vi "Dashboard Main.vi"() -> ()   [LabVIEW 2015]
uses:
  Auton Defenses Enum.ctl
  AutoStatesTypeDef.ctl
  <vilib>/Utility/miscctls.llb/LVRowAndColumnTypeDef.ctl
  <vilib>/event_ctls.llb/eventvkey.ctl
  <vilib>/Rock Robotics/WPI/Dashboard/WPI_DashboardLogging Global.vi
  <vilib>/Rock Robotics/Network Tables/NT Read Numeric Array.vi
  <vilib>/Rock Robotics/Network Tables/NT Write Boolean.vi
  <vilib>/Rock Robotics/Network Tables/NT Read Boolean.vi
  <vilib>/Rock Robotics/Network Tables/NT Write Numeric Array.vi
  <vilib>/Utility/config.llb/Write Key (String).vi
  <vilib>/Utility/config.llb/Write Key (I32).vi
  <vilib>/Utility/config.llb/NI_LVConfig.lvlib
panel:
  in  "End Point 2":cluster{"X":i32, "Y":i32}={"X"=158, "Y"=0}
  in  "Start Point 2":cluster{"X":i32, "Y":i32}={"X"=158, "Y"=240}
  in  "End Point":cluster{"X":i32, "Y":i32}={"X"=320, "Y"=120}
  in  "Start Point":cluster{"X":i32, "Y":i32}={"X"=0, "Y"=120}
  in  "Vision":u16(ring) items=["Camera Off", "USB Camera SW", "USB Camera HW", "IP Camera"]
  out "Detected Targets":T1(array[cluster]) {"Normalized Rect"."Numeric 5" format="%#_2g"; "Normalized Rect"."Numeric 3" format="%#_2g"; "Normalized Rect"."Numeric 2" format="%#_2g"; "Normalized Rect"."Numeric" format="%#_2g"}
  in  "TCP":refnum<k5>
  in  "Rec Mode":enum32{"Stop", "Record", "Playback"}(radio)
  out "Camera IP":string
  out "Image Message":string="Timeout in Camera Communications"
  in  "Dashboard Tab":T2(tab)
  out "Shooter at Speed":bool
  in  "Right Compensation":dbl
  in  "Left Compensation":dbl
  out "Rear Camera On?":bool
  out "Drive Shift":string
  out "Gyro Angle":dbl
  out "Drive Mode":string
  out "Shooter Speed":dbl
  out "Shooter Setpoint":dbl
  out "Hanging Pin Status":string
  out "Ball on Board?":bool
  in  "Defense":T3
  in  "Position":T4(ring)
  in  "Enable Vision?":bool
  out "Shooter Active?":bool
  in  "Gyro Reset":bool
  out "Acquiring?":bool
  out "Auton Current State":T5
  in  "Auton Shoot":bool
  in  "Select Auto":string(combo)
  out "NT Connection":bool
  in  "Camera Settings":T6={"Frame Rate"=30, "Compression"=30, "Size"=1} {"Frame Rate" scale=1.0..30.0; "Size" items=["640x480", "320x240", "160x120"]}
  out "MotorChart R":cluster{"Numeric":dbl, "Numeric":dbl}(graph)
  out "MotorChart L":T7(graph)
  out "MotorSliders R":cluster{"MotorSlide1":dbl, "MotorSlide2":dbl} {"MotorSlide2" scale=-1.0..1.0 scale format="%#_2e"; "MotorSlide1" scale=-1.0..1.0 scale format="%#_2e"}
  out "MotorSliders L":T8 {"MotorSlide4 2" scale=0.0..14.0 scale format="%#_2e"; "MotorSlide2" scale=-1.0..1.0 scale format="%#_2e"; "MotorSlide1" scale=-1.0..1.0 scale format="%#_2e"}
  out "Gyro":dbl(knob) scale=0.0..360.0
  out "JS1 Z":dbl(slide) scale=-1.0..1.0 scale format="%#_2e"
  out "JS1 Graph":cluster{"X":dbl, "Y":dbl}[](graph)
  out "JS1 Buttons":T9
  out "JS2 Z":dbl(slide) scale=-1.0..1.0 scale format="%#_2e"
  out "JS2 Graph":cluster{"X":dbl, "Y":dbl}[](graph)
  out "JS2 Buttons":T9
  out "Mode":T10(ring)=enum."Auto Disabled"
  in  "DB Camera Config":bool
  out "fps":dbl format="%#.1g"
  out "Mbps":dbl format="%#.1g"
  out "Mbps LED":bool
  in  "DB/String 9":string
  in  "DB/String 8":string
  in  "DB/String 7":string
  in  "DB/String 6":string
  in  "DB/String 5":string
  in  "DB/String 4":string
  in  "DB/String 3":string
  in  "DB/String 2":string
  in  "DB/String 1":string
  in  "DB/String 0":string
  in  "DB/Slider 0":dbl(slide) scale=0.0..5.0
  in  "DB/Slider 1":dbl(slide) scale=0.0..5.0
  in  "DB/Slider 2":dbl(slide) scale=0.0..5.0
  in  "DB/Slider 3":dbl(slide) scale=0.0..5.0
  out "DB/LED 3":bool
  out "DB/LED 2":bool
  out "DB/LED 1":bool
  out "DB/LED 0":bool
  in  "DB/Button 3":bool
  in  "DB/Button 2":bool
  in  "DB/Button 1":bool
  in  "DB/Button 0":bool caption="New Name"
  in  "Shooter Control":bool=TRUE
  in  "Top Wheel Speed Multiplier":dbl=0.8
  in  "Beater Bar Speed":dbl=0.75
  in  "LED Color":T11={"Hue"={77.0, 147.0}, "Sat"={140.0, 255.0}, "Val"={146.0, 255.0}} {"Hue" scale=0.0..255.0 scale format="%#_3g"}
  out "Target X Value":dbl
  in  "Shooter Power":dbl=0.5 step=0.01
  out "Shooter Speed (RPS)":dbl
  in  "Shooter Setpoint (RPS)":dbl=49.0 step=0.01
  in  "Shooter Wait (Seconds)":dbl=0.75 step=0.01
  out "Shooter Speed Top (RPS)":dbl
  in  "Test Slider":dbl(slide) scale=0.0..100.0 scale format="%#_3g"
  in  "On/Off":bool caption="Solenoid"
  in  "Test Name":u16(ring) items=["Select the test to run..."]
  in  "Test Tree":string(tree)
  in  "Motor":cluster{"Value":dbl, "Enable":bool} {"Value" scale=-1.0..1.0 scale format="%#_3g"}
  out "Progress":T12 {"Test Progress" scale=0.0..100.0}
  in  "Rev/Fwd":cluster{"Forward":bool, "Reverse":bool}
  in  "Test Ring":u16(ring) items=["Monochrome", "Color"]
  out "Cmd Status":string
  in  "Execute Command":bool
  in  "Command Params":string[][](table)
  in  "Command Selection":i32(listbox)
  in  "CheckList":i32(listbox)
  out "Tree":string(tree)
  out "Background":bool
  out "Unmasked Image":T13(plugin-control)
  # "Adds to specified,\nsubtracts from other(-1 to 1)"
  # "Left"
  # "Front"
  # "Right"
  # "Battery"
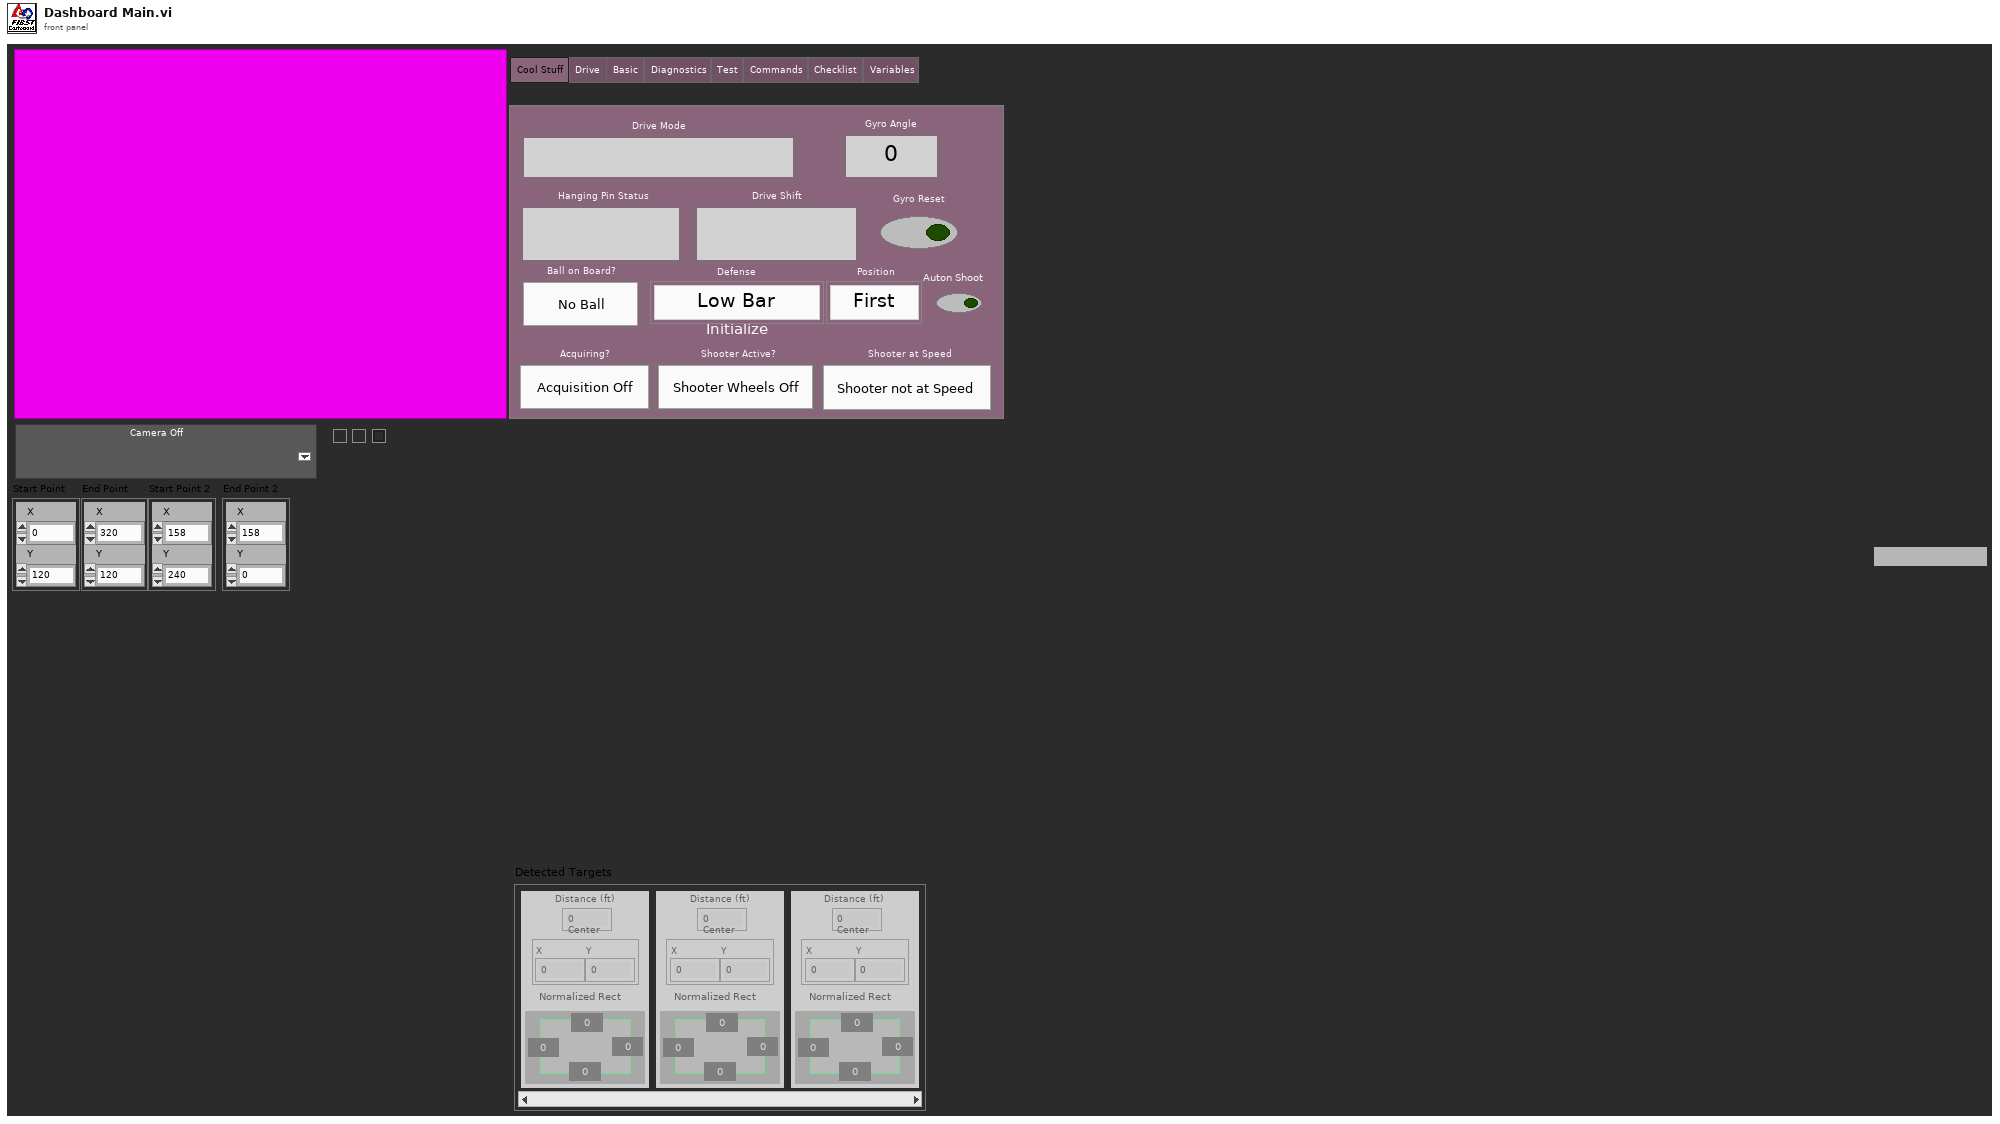
[diagram p1: front panel]
types:
  T1 = cluster{"Distance (ft)":dbl, "Center":cluster{"X":dbl, "Y":dbl}, "Normalized Rect":cluster{"Numeric":dbl, "Numeric 2":dbl, "Numeric 3":dbl, "Numeric 5":dbl}}[]
  T2 = enum32{"Cool Stuff", "Drive", "Basic", "Diagnostics", "Test", "Commands", "Checklist", "Variables"}
  T3 = typedef "Auton Defenses Enum.ctl" = enum16{"Low Bar", "None", "Portcullis", "CDF", "Moat", "Ramparts", "Drawbridge", "Sally Port", "Rock Wall", "Reach", "Spy Bot", "Rough Terrain"}
  T4 = enum16{"First", "Second", "Third", "Fourth", "Fifth"}
  T5 = typedef "AutoStatesTypeDef.ctl" = enum16{"Initialize", "Line up to shoot", "Align robot", "Drive to goal", "Lower Arms", "Raise Arms", "Drive to defense", "Cross defense", "Turn towards goal", "Shoot", "Retreat", "Stop"}
  T6 = cluster{"Frame Rate":i32, "Compression":i32, "Size":u16}
  T7 = cluster{"Numeric":dbl, "Numeric":dbl, "Battery V":dbl}
  T8 = cluster{"MotorSlide1":dbl, "MotorSlide2":dbl, "MotorSlide4 2":dbl}
  T9 = cluster{bool, bool, bool, bool, bool, bool, bool, bool, bool, bool, bool, bool}
  T10 = enum8{"Tele-Op Disabled", "Tele-Op Enabled", "Auto Disabled", "Auto Enabled", "Test Disabled", "Test Enabled", "Disconnected", "No Code", "E-Stop"}
  T11 = cluster{"Hue":cluster{dbl, dbl}, "Sat":cluster{dbl, dbl}, "Val":cluster{dbl, dbl}}
  T12 = cluster{"Test Progress":u8, "Test Progress Text":string}
  T13 = typedef "IMAQ Image.ctl" = refnum<image>
  T14 = cluster{"IDs":cluster{"RPC field ID":u16, "Unique ID":u16}, "String":string}
  T15 = enum32{"Drive", "Basic", "Custom", "Test", "Checklist", "Variables"}
  T16 = typedef "Image Type" = u32
  T17 = cluster{"Unmasked Image":refnum<vi>, "Dashboard Tab":refnum<vi>, "Background":refnum<vi>, "Vision":refnum<vi>, "Rec Mode":refnum<vi>, "Test Slider":refnum<vi>, "On/Off ":refnum<vi>, "Test Ring":refnum<vi>, "Rev/Fwd":refnum<vi>, "Test Name":refnum<vi>, "Motor":refnum<vi>, "Progress":refnum<vi>, "CheckList":refnum<vi>, "Tree":refnum<vi>, "Test Tree":refnum<vi>, "Command Params":refnum<vi>, "Command Selection":refnum<vi>, "Execute Command":refnum<vi>, "Cmd Status":refnum<vi>}
  T18 = typedef "NI_LVConfig.lvlib/Config Data RefNum.ctl" = refnum<k1>
  T19 = cluster{"Distance (ft)":dbl, "Center":cluster{dbl, dbl}, "Normalized Rect":cluster{"Numeric":dbl, "Numeric 2":dbl, "Numeric 3":dbl, "Numeric 5":dbl}}[]
  T20 = cluster{"Error Strings":string, "Disable Counts":cluster{u16, u16}, "Rail Faults":cluster{u16, u16, u16}, "Robot IP":string, "DB Mode":u8, "Event Info":cluster{"Name":string, "Type":u8, "Number":u16, "Replay":u8}, "Camera Addr":string}
  T21 = cluster{"Storage":cluster{"Disk Free":u64, "RAM Block":u32, "RAM free":u32}, "CPU Utilization":cluster{"CPU % ISR":sgl, "CPU % Time Crit":sgl, "CPU % Timed Str":sgl, "CPU % High":sgl, "CPU % Above":sgl, "CPU % Normal":sgl, "CPU % Low":sgl}, "CAN":cluster{"% Bus Utilization":sgl, "Bus Off Cnt":u32, "TX_FIFO Full Cnt":u32, "Receive Error Cnt":u8, "Transmit Error Cnt":u8}, "HID":cluster{"HID Outputs":u32, "Rumble Low":u16, "Rumble High":u16}[]}
  T22 = cluster{"Status bits":cluster{"Test Mode":bool, "Autonomous":bool, "Enabled":bool, "Code Start":bool, "Brownout":bool, "Reserved 2":bool, "Reserved 3":bool, "E-Stop":bool}, "Code Trace":cluster{"Disabled":bool, "TeleOp":bool, "Auto":bool, "Test":bool}, "Controller Type":enum16{"unknown", "cRIO", "roboRio"}, "Code?":enum16{"unknown", "noCode", "code"}, "Battery V":dbl}
  T23 = cluster{"Control Bits":cluster{"TestMode":bool, "Autonomous":bool, "Enabled":bool, "FMS Present":bool, bool, bool, bool, "E-Stop":bool}, "Team Station ":u8, "Countdown":sgl, "Joystick Values":cluster{"Axes":dbl[], "Buttons":bool[], "POVs":i16[]}[]}
  T24 = cluster{"Axes":dbl[], "Buttons":bool[], "POVs":i16[]}[]
  T25 = cluster{"Distance (ft)":dbl, "Center":cluster{"X":dbl, "Y":dbl}, "Normalized Rect":cluster{"Numeric":dbl, "Numeric 2":dbl, "Numeric 3":dbl, "Numeric 5":dbl}}
  T26 = cluster{"Axes":dbl[], "Buttons":bool[], "POVs":i16[]}
  T27 = cluster{"Buttons[0]":bool, "Buttons[1]":bool, "Buttons[2]":bool, "Buttons[3]":bool, "Buttons[4]":bool, "Buttons[5]":bool, "Buttons[6]":bool, "Buttons[7]":bool, "Buttons[8]":bool, "Buttons[9]":bool, "Buttons[10]":bool, "Buttons[11]":bool}
  T28 = cluster{"Operation":enum16{"Update", "Clear"}, "Color Box":u32}[]
  T29 = typedef "eventvkey.ctl" = enum16{"ASCII", "Enter", "Return", "Shift", "Ctrl", "Alt", "Cmd", "Opt", "Caps", "NumLock", "Clear", "Break", "Up", "Down", "Left", "Right", "Insert", "Delete", "Home", "End", "PageUp", "PageDown", "Escape", "Help", "Pause", "ScrollLock", "F1", "F2", "F3", "F4", "F5", "F6", "F7", "F8", "F9", "F10", "F11", "F12", "F13", "F14", "F15", "F16", "F17", "F18", "F19", "F20", "F21", "F22", "F23", "F24", "Play", "VolumeUp", "VolumeDown", "Mute", "Two Byte Char"}
  T30 = cluster{"Image Size":bool, "Image Type":bool, "Pixel Value":bool, "ROI Information":bool, "Zoom Factor":bool}
  T31 = enum8{"Enabled", "Disabled", "Disabled and Grayed Out"}
  T32 = cluster{"Operation":enum16{"Update", "Clear"}, "Color Box":u32}
  T33 = typedef "LVRowAndColumnTypeDef.ctl" = cluster{"Row":i32, "Column":i32}
  T34 = cluster{"Shift":bool, "Ctrl":bool, "Alt":bool, "Cmd":bool, "Opt":bool}
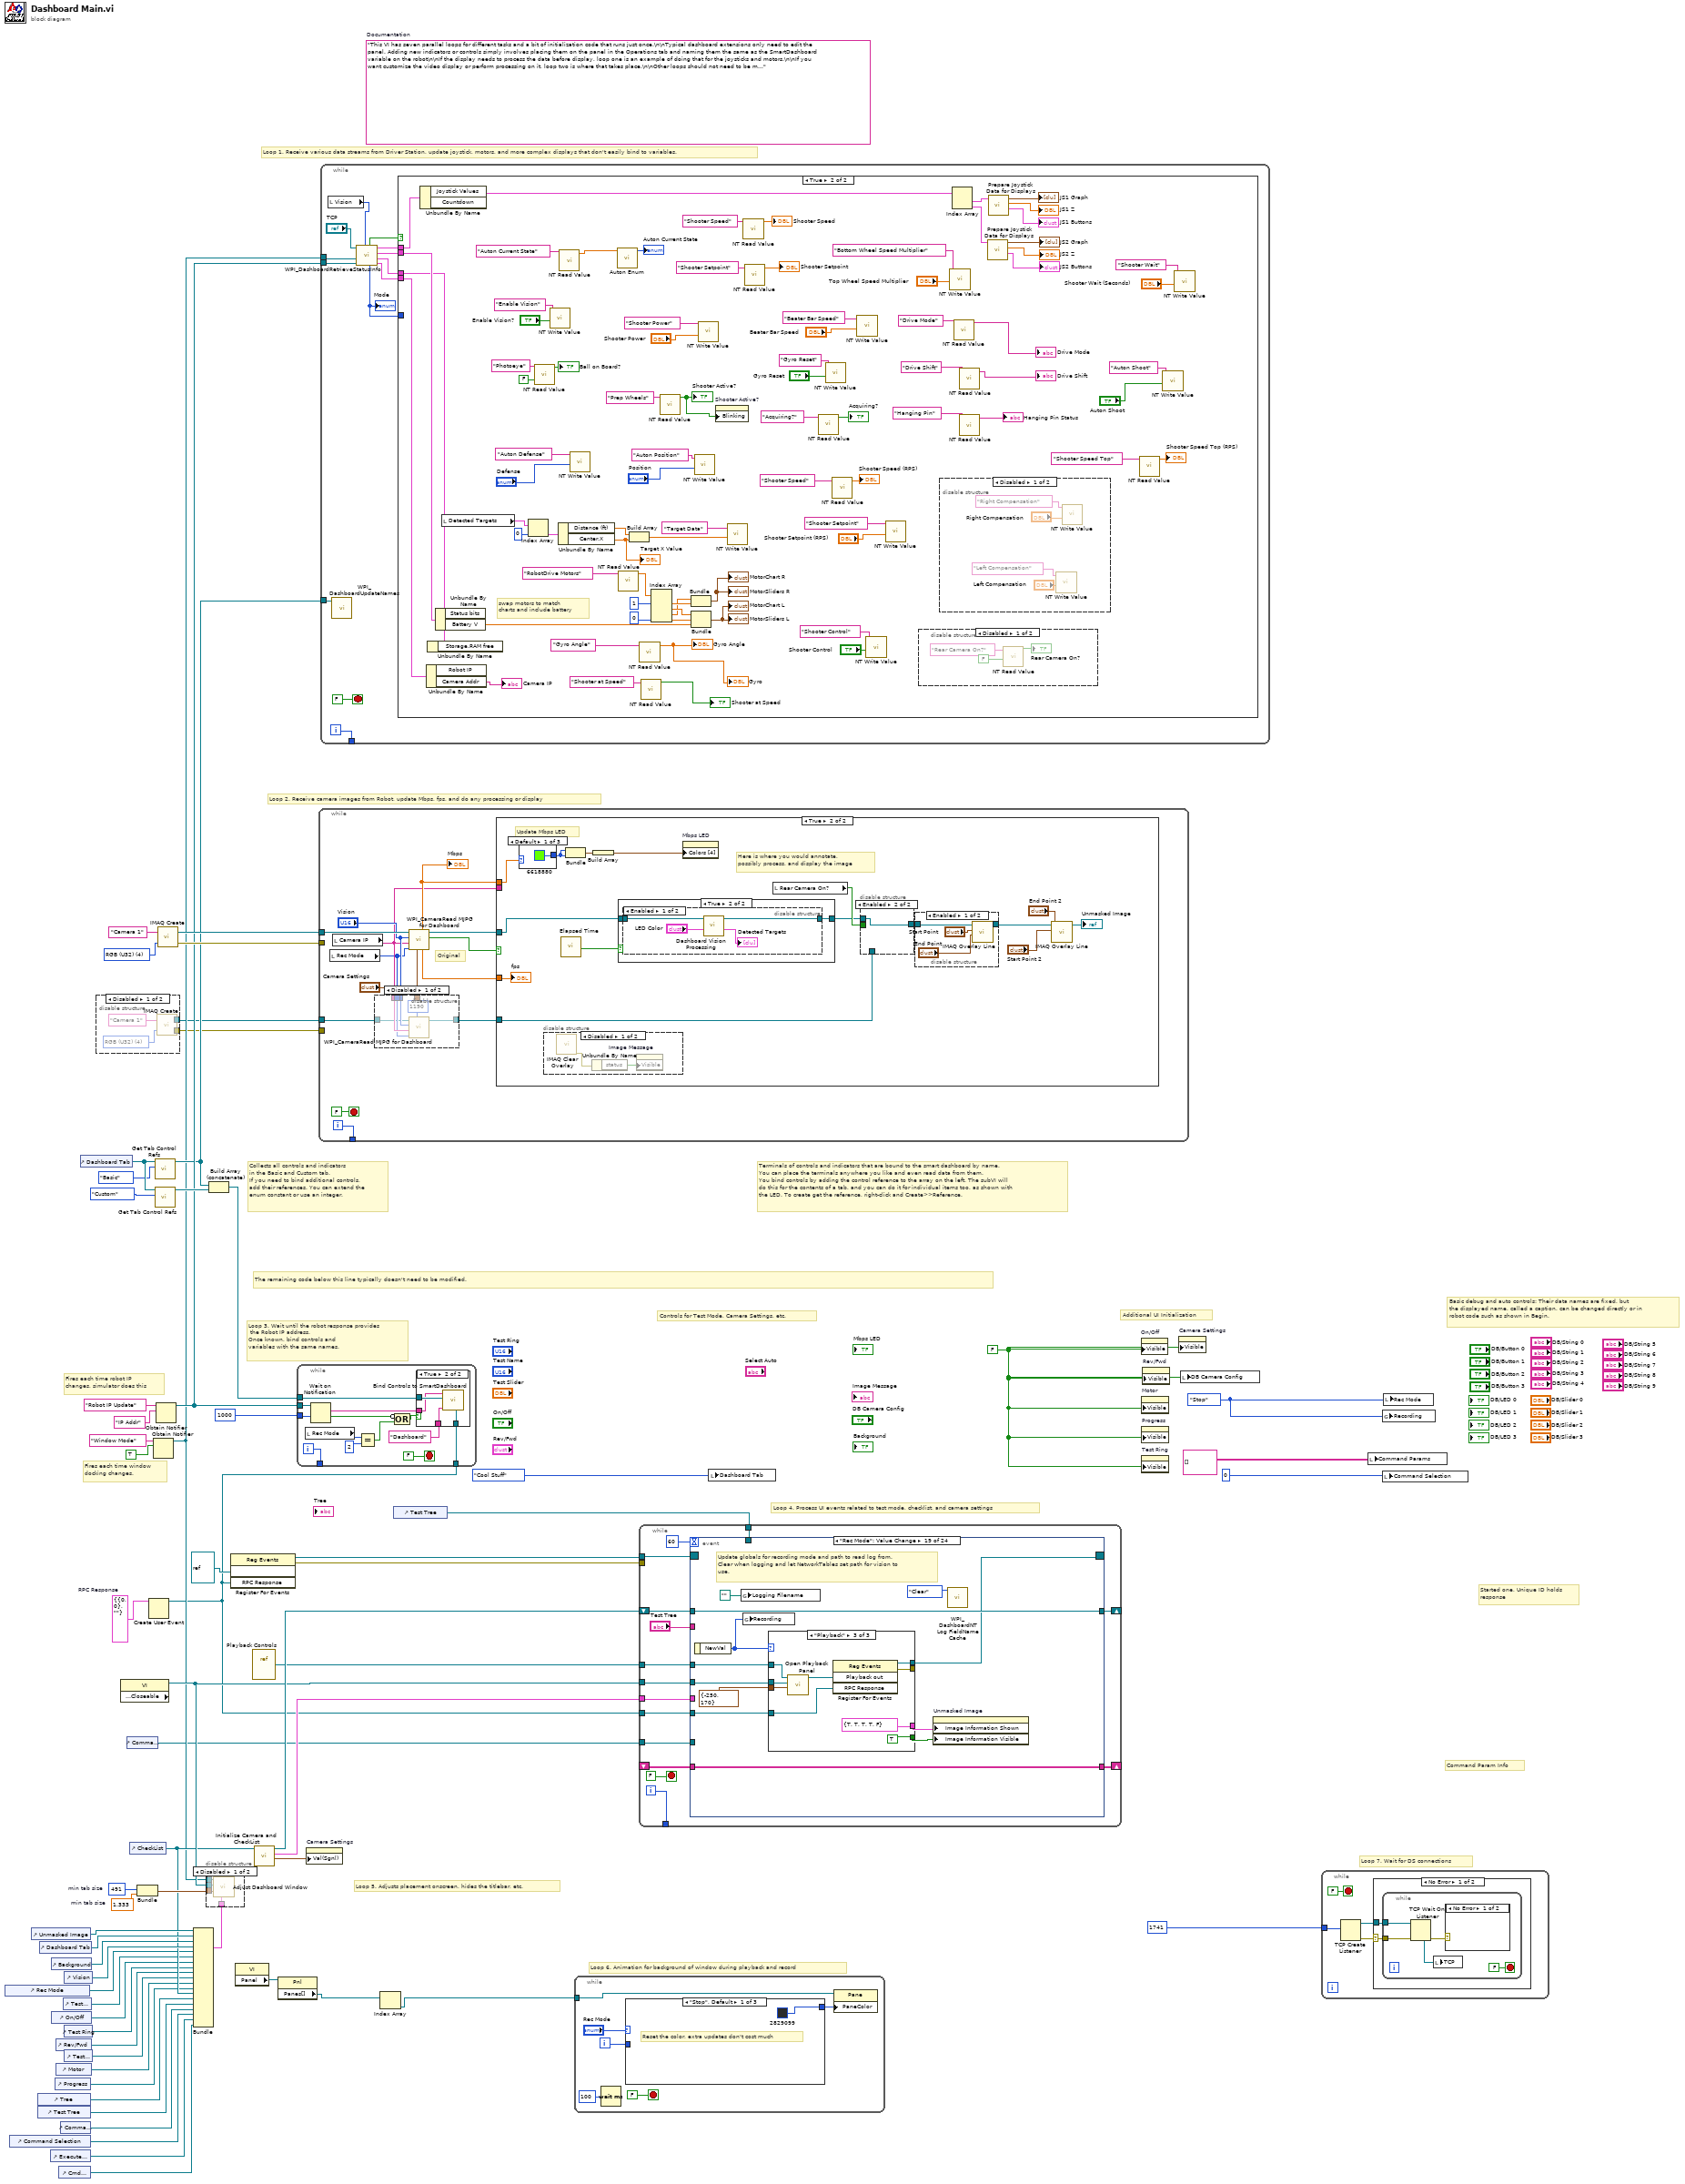
[diagram p0: block diagram]
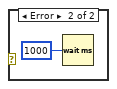
[diagram p4: hidden frame]
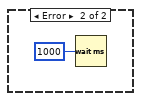
[diagram p5: hidden frame]
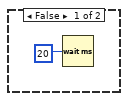
[diagram p6: hidden frame]
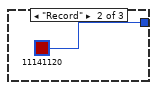
[diagram p9: hidden frame]
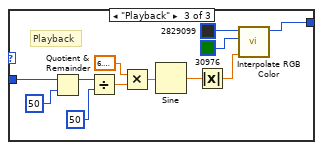
[diagram p10: hidden frame]
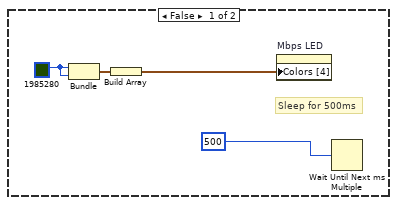
[diagram p13: hidden frame]
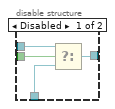
[diagram p17: hidden frame]
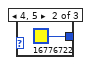
[diagram p19: hidden frame]
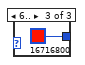
[diagram p20: hidden frame]
diagram:
  w9 = T14 {"IDs"={"RPC field ID"=0, "Unique ID"=0}, "String"=""}  # RPC Response
  w35 = 491  # min tab size
  w34 = 1.333  # min tab size
  w43 = enum32{"Stop", "Record", "Playback"}."Stop" ("Rec Mode")
  w17 = FALSE ("Visible")
  (unwired) "This VI has seven parallel loops for different tasks and a bit of initialization code that runs just once.\n\nTypical dashboard extensions only need to edit the panel. Adding new indicators or controls simply involves placing them on the panel in the Operations tab and naming them the same as the SmartDashboard variable on the robot\n\nIf the display needs to process the data before display, loop one is an example of doing that for the joysticks and motors.\n\nIf you want customize the video display or perform processing on it, loop two is where that takes place.\n\nOther loops should not need to be modified. They are pretty standard, and document the task they perform."  # Documentation
  w63 = T16 4 items=["Grayscale (U8)", "Grayscale (I16)", "Grayscale (SGL)", "Complex (CSG)", "RGB (U32)", "HSL (U32)", "RGB (U64)"] ("Image Type")
  # "Command Param Info"
  # "Started one, Unique ID holds\nresponse"
  # "Loop 7. Wait for DS connections"
  # "Basic debug and auto controls: Their data names are fixed, but\nthe displayed name, called a caption, can be changed directly or in\nrobot code such as shown in Begin."
  # "Controls for Test Mode, Camera Settings, etc."
  # "Additional UI Initialization"
  # "Loop 6. Animation for background of window during playback and record"
  # "Fires each time robot IP\nchanges, simulator does this"
  # "Fires each time window\ndocking changes."
  # "Collects all controls and indicators\nin the Basic and Custom tab.\nIf you need to bind additional controls,\nadd their references. You can extend the\nenum constant or use an integer."
  # "The remaining code below this line typically doesn't need to be modified."
  # "Loop 4. Process UI events related to test mode, checklist, and camera settings"
  # "Terminals of controls and indicators that are bound to the smart dashboard by name.\nYou can place the terminals anywhere you like and even read data from them.\nYou bind controls by adding the control reference to the array on the left. The subVI will\ndo this for the contents of a tab, and you can do it for individual items too, as shown with\nthe LED. To create get the reference, right-click and Create>>Reference."
  # "Loop 3. Wait until the robot response provides\n the Robot IP address.\nOnce known, bind controls and\nvariables with the same names."
  # "Loop 5. Adjusts placement onscreen, hides the titlebar, etc."
  # "Loop 1. Receive various data streams from Driver Station, update joystick, motors, and more complex displays that don't easily bind to variables."
  # "Loop 2. Receive camera images from Robot, update Mbps, fps, and do any processing or display"
  n1 = control-ref of="Rec Mode"() -> (w23:refnum<vi>)
  n2 = control-ref of="Command Selection"() -> (w8:refnum<vi>)
  n3 = control-ref of="Unmasked Image"() -> (w38:refnum<vi>)
  n4 = control-ref of="Tree"() -> (w27:refnum<vi>)
  n5 = control-ref of="Test Tree"() -> (w26:refnum<vi>)
  n6 = control-ref of="Dashboard Tab"() -> (w37:refnum<vi>)
  n7 = control-ref of="Execute Command"() -> (w10:refnum<vi>)
  n8 = control-ref of="Background"() -> (w32:refnum<vi>)
  n9 = control-ref of="On/Off"() -> (w21:refnum<vi>)
  n10 = control-ref of="Progress"() -> (w18:refnum<vi>)
  n11 = control-ref of="Rev/Fwd"() -> (w19:refnum<vi>)
  n12 = control-ref of="Motor"() -> (w24:refnum<vi>)
  n13 = control-ref of="Cmd Status"() -> (w4:refnum<vi>)
  n14 = control-ref of="Command Params"() -> (w11:refnum<vi>)
  n15 = control-ref of="Test Slider"() -> (w22:refnum<vi>)
  n16 = control-ref of="Vision"() -> (w36:refnum<vi>)
  n17 = control-ref of="Test Ring"() -> (w20:refnum<vi>)
  n18 = control-ref of="Test Name"() -> (w25:refnum<vi>)
  n19 = control-ref of="Dashboard Tab"() -> (w41:refnum<vi>)
  n20 = disable-structure shown="Disabled" {
    disable-tunnel: [w65 _] -> w2
    disable-tunnel: [w64 _] -> w1
    frame Disabled {
      w66 = T16 4 items=["Grayscale (U8)", "Grayscale (I16)", "Grayscale (SGL)", "Complex (CSG)", "RGB (U32)", "HSL (U32)", "RGB (U64)"] ("Image Type")
      n21 = call "IMAQ Create"("Image Name"="Camera 1", "Image Type"=w66) -> ("New Image"=w65:T13, "error out"=w64:errorcluster)  [unwired: 2 in, 1 out]
    }
    frame Enabled {
    }
  }
  n22 = property class="VI" props=["Front Panel.Closeable"]() -> (reference out=w42:refnum<vi>)  [unwired: 2 in, 2 out]
  n23 = control-ref of="Command Params"() -> (w3:refnum<vi>)
  n24 = control-ref of="CheckList"() -> (w28:refnum<vi>)
  n25 = Bundle("min tab size"=w35, "min tab size"=w34) -> (w33:cluster{"min tab size":i32, "min tab size":dbl})  [unwired: 1 in]
  n26 = Create User Event(user event datatype=w9) -> (user event=w5:refnum<user-event>)  [unwired: 1 in, 1 out]
  n27 = Obtain Notifier(name (unnamed)="Window Mode", notification data type=TRUE) -> (notifier out=w14:refnum<notifier>)  [unwired: 2 in, 2 out]
  n28 = call <vilib>:"Get Tab Control Refs.vi"("Page Index"=T15."Basic" ("Dashboard Tab"), "TabControl in"=w41) -> ("ControlsOnPage"=w15:refnum<vi>[])  [unwired: 9 in]
  n29 = call <vilib>:"Get Tab Control Refs.vi"("Page Index"=T15."Custom" ("Dashboard Tab"), "TabControl in"=w41) -> ("ControlsOnPage"=w40:refnum<vi>[])  [unwired: 9 in]
  n30 = Obtain Notifier(name (unnamed)="Robot IP Update", notification data type="IP Addr" ("name (unnamed)")) -> (notifier out=w16:refnum<notifier>)  [unwired: 2 in, 2 out]
  n31 = call "IMAQ Create"("Image Name"="Camera 1", "Image Type"=w63) -> ("New Image"=w61:T13, "error out"=w60:errorcluster)  [unwired: 2 in, 1 out]
  n32 = Bundle("Unmasked Image"=w38, "Dashboard Tab"=w37, "Background"=w32, "Vision"=w36, "Rec Mode"=w23, "Test Slider"=w22, "On/Off"=w21, "Test Ring"=w20, "Rev/Fwd"=w19, "Test Name"=w25, "Motor"=w24, "Progress"=w18, "CheckList"=w28, "Tree"=w27, "Test Tree"=w26, "Command Params"=w11, "Command Selection"=w8, "Execute Command"=w10, "Cmd Status"=w4) -> (w29:T17)  [unwired: 1 in]
  n33 = disable-structure shown="Disabled" {
    disable-tunnel: w42 -> [w71 _]
    disable-tunnel: w33 -> [w70 _]
    disable-tunnel: w29 -> [w69 _]
    disable-tunnel: w14 -> [w68 _]
    frame Disabled {
      n34 = call "Adjust Dashboard Window.vi"("Sizing Refnums"=w69, "Size Constraints"=w70, "VI"=w71, "WIn Mode"=w68) -> ()  [unwired: 8 in]
    }
    frame Enabled {
    }
  }
  n35 = Build Array (concatenate)(w15, w40) -> (w39:refnum<vi>[])
  n36 = register-events(refnum<vi> refnum, w5) -> (reference out=w47:refnum<event-registration>, error out=w46:errorcluster)  [unwired: 2 in]
  n37 = property class="VI"() -> ("Panel"=w50:refnum<vi>)  [unwired: 2 in, 2 out]
  n38 = vi-ref "Playback Controls.vi"() -> (w48:refnum<vi>)
  n39 = call "Initialize Camera and CheckList.vi"("ListBox in"=w28) -> ("Cluster"=w54:cluster{"value":i32, "value":i32, "index":i32}, "Array"=w55:cluster{string[]}[], "File Refnum"=w53:T18)  [unwired: 8 in]
  n40 = property class="Pnl"(reference=w50) -> ("Panes[]"=w51:refnum<vi>[])  [unwired: 1 in, 2 out]
  n41 = while {
    tunnel: w39 -> [w84]
    tunnel: w16 -> [w82]
    tunnel: [w80] -> _
    tunnel: u32 1000 ("milliseconds to wait") -> [w79]
    tunnel: w5 -> [w72]
    i -> [w80]
    stop <- FALSE stop-if-true
    n42 = local read "Rec Mode"() -> (w75:enum32{"Stop", "Record", "Playback"})
    n43 = Wait on Notification(notifier=w82, timeout in ms (-1)=w79) -> (notification=w81:string, timed out?=w77:bool)  [unwired: 2 in, 2 out]
    n44 = Equal?(x=w75, y=u16 2 ("Rec Mode")) -> (x = y?=w76:bool)
    n45 = Compound Arithmetic op=OR(invert w77, w76) -> (w78:bool)
    n46 = case shown="True" w78 {
      tunnel: w84 -> [_ w88]
      tunnel: w81 -> [_ w87]
      tunnel: "Dashboard" -> [_ w86]
      tunnel: w72 -> [_ w85]
      frame False {
      }
      frame True {
        n47 = call <vilib>:"Bind Controls to SmartDashboard.vi"("RPC ref"=w85, "Client Name"=w86, "Bound Control Refs"=w88, "Server IP Address"=w87) -> ()  [unwired: 8 in]
      }
    }
  }
  n48 = property on="Camera Settings" class="Clust (strict)"("Val(Sgnl)"=w54) -> ()  [unwired: 2 in, 2 out]
  n49 = while {
    tunnel: w60 -> [_]
    tunnel: [w100] -> _
    tunnel: w61 -> [w99]
    tunnel: w2 -> [w89]
    tunnel: w1 -> [_]
    i -> [w100]
    stop <- FALSE stop-if-true
    # "Original"
    n50 = local read "Rec Mode"() -> (w92:enum32{"Stop", "Record", "Playback"})
    n51 = local read "Camera IP"() -> (w93:string)
    n52 = disable-structure shown="Disabled" {
      disable-tunnel: "Vision" -> [w107 _]
      disable-tunnel: w93 -> [w106 _]
      disable-tunnel: w92 -> [w105 _]
      disable-tunnel: [w104 _] -> w91
      disable-tunnel: "Camera Settings" -> [w103 _]
      disable-tunnel: w89 -> [w102 _]
      frame Disabled {
        n53 = call <vilib>:"WPI_CameraRead MJPG for Dashboard.vi"("Camera Settings"=w103, 7:u16 1190 ("port"), "Rec Mode"=w105, "Camera IP"=w106, "Camera Mode"=w107, "Refnum in"=w102) -> ("Refnum out"=w104:T13)  [unwired: 2 in, 3 out]
      }
      frame Enabled {
      }
    }
    n54 = call <vilib>:"WPI_CameraRead MJPG for Dashboard.vi"("Camera Settings"="Camera Settings", "Rec Mode"=w92, "Camera IP"=w93, "Camera Mode"="Vision", "Refnum in"=w99) -> ("Active"=w95:bool, "Refnum out"=w98:T13, "FPS"=w97:dbl, "Bandwidth (Mbps)"=w96:dbl)  [unwired: 3 in]
    "Mbps" <- w96
    n55 = case shown="True" w95 {
      tunnel: w98 -> [_ w121]
      tunnel: w96 -> [_ w124]
      tunnel: w97 -> [_ w123]
      tunnel: w93 -> [_ _]
      tunnel: w91 -> [_ w119]
      frame False {
        w109 = u32 1985280 ("Color Box")
        # "Sleep for 500ms"
        n56 = Bundle("Color Box"=w109, "Color Box"=w109) -> (w111:cluster{"Color Box":u32, "Color Box":u32})  [unwired: 1 out]
        n57 = Build Array(w111) -> (w110:cluster{"Color Box":u32, "Color Box":u32}[])
        n58 = property on="Mbps LED" class="Bool (strict)"("Colors [4]"=w110) -> ()  [unwired: 2 in, 2 out]
        n59 = Wait Until Next ms Multiple(millisecond multiple=u32 500) -> ()  [unwired: 1 out]
      }
      frame True {
        # "Here is where you would annotate,\npossibly process, and display the image"
        # "Update Mbps LED"
        n60 = case shown="Default" w124 {
          tunnel: [u32 6618880 ("Color Box") u32 16776722 ("Color Box") u32 16716800 ("Color Box")] -> w125
          frame Default {
          }
          frame 4, 5 {
          }
          frame 6.. {
          }
        }
        n61 = disable-structure shown="Disabled" {
          frame Disabled {
            n62 = call "IMAQ Clear Overlay"() -> ("error out"=w146:errorcluster)  [unwired: 3 in, 8 out]
            n63 = Unbundle By Name(w146) -> ("status"=w147:bool)
            n64 = property on="Image Message" class="Str"("Visible"=w147) -> ()  [unwired: 2 in, 2 out]
          }
          frame Enabled {
          }
        }
        n65 = call "Elapsed Time"() -> ("Time has Elapsed"=w118:bool)  [unwired: 12 in, 7 out]
        n66 = Bundle("Color Box"=w125, "Color Box"=w125) -> (w127:cluster{"Color Box":u32, "Color Box":u32})  [unwired: 1 out]
        n67 = Build Array(w127) -> (w126:cluster{"Color Box":u32, "Color Box":u32}[])
        n68 = case shown="True" w118 {
          tunnel: w121 -> [w133 w135]
          tunnel: [w133 w134] -> w120
          frame False {
          }
          frame True {
            n69 = disable-structure shown="Enabled" {
              disable-tunnel: w135 -> [w139 w140]
              disable-tunnel: [w138 w140] -> w134
              frame Enabled {
                n70 = call "Dashboard Vision Processing.vi"("LED Color"="LED Color", "Camera Image"=w139) -> ("Detected Targets"=→"Detected Targets":T19, "Orig Image"=w138:T13)  [unwired: 8 in]
              }
              frame Disabled {
              }
            }
          }
        }
        n71 = property on="Mbps LED" class="Bool (strict)"("Colors [4]"=w126) -> ()  [unwired: 2 in, 2 out]
        n72 = local read "Rear Camera On?"() -> (w122:bool)
        n73 = disable-structure shown="Enabled" {
          disable-tunnel: w122 -> [w144 _]
          disable-tunnel: [w143 w145] -> w117
          disable-tunnel: w120 -> [w142 w145]
          disable-tunnel: w119 -> [w141 _]
          frame Disabled {
            n74 = Select(t=w142, s=w144, f=w141) -> (s? t:f=w143:T13)
          }
          frame Enabled {
          }
        }
        n75 = disable-structure shown="Enabled" {
          disable-tunnel: w117 -> [w131 w132]
          disable-tunnel: [w130 w132] -> w115
          frame Enabled {
            n76 = call "IMAQ Overlay Line"("End Point"="End Point", "Start Point"="Start Point", "Image"=w131) -> ("Image Out"=w130:T13)  [unwired: 7 in, 1 out]
          }
          frame Disabled {
          }
        }
        n77 = call "IMAQ Overlay Line"("End Point"="End Point 2", "Start Point"="Start Point 2", "Image"=w115) -> ("Image Out"=→"Unmasked Image":T13)  [unwired: 7 in, 1 out]
        "fps" <- w123
      }
    }
  }
  n78 = while {
    tunnel: [w162] -> _
    tunnel: w16 -> [w156]
    tunnel: w15 -> [w155]
    tunnel: w14 -> [w151]
    i -> [w162]
    stop <- FALSE stop-if-true
    n79 = local read "Vision"() -> (w153:u16)
    n80 = call <vilib>:"WPI_DashboardUpdateNames.vi"("Controls on Tab"=w155) -> ()  [unwired: 11 in]
    n81 = call <vilib>:"WPI_DashboardRetrieveStatusInfo.vi"("Vision"=w153, "Binding Refnum"=w156, "Window Mode Notifier"=w151, "TCP Cnx"="TCP") -> ("Power and Errors"=w157:T20, "Robot Metrics"=w160:T21, "Status Info"=w161:T22, "Control Info"=w158:T23, "Robot Mode"=w154:T10, "Process?"=w159:bool)  [unwired: 2 in]
    "Mode" <- w154
    n82 = case shown="True" w159 {
      tunnel: w161 -> [_ w246]
      tunnel: w160 -> [_ w245]
      tunnel: w158 -> [_ w244]
      tunnel: w157 -> [_ w243]
      tunnel: w154 -> [_ _]
      frame False {
        n83 = Wait (ms)(milliseconds to wait=u32 20) -> ()  [unwired: 1 out]
      }
      frame True {
        # "swap motors to match\ncharts and include battery"
        n84 = Unbundle By Name(w244) -> ("Joystick Values"=w233:T24)  [unwired: 1 out]
        n85 = Unbundle By Name(w243) -> ("Camera Addr"=→"Camera IP":string)  [unwired: 1 out]
        n86 = Unbundle By Name(w245) -> ()  [unwired: 1 out]
        n87 = Unbundle By Name(w246) -> ("Battery V"=w234:dbl)  [unwired: 1 out]
        n88 = local read "Detected Targets"() -> (w207:T1)
        n89 = Index Array(array=w207, index=0) -> (element=w205:T25)
        n90 = call-poly <vilib>:"NT Read Value.vi"("Default Value"=FALSE, "Name"="Photoeye") -> ("Boolean"=→"Ball on Board?":bool)  [unwired: 8 in, 1 out]
        n91 = call-poly <vilib>:"NT Write Value.vi"("Boolean"="Enable Vision?", "Name"="Enable Vision") -> ()  [unwired: 9 in, 1 out]
        n92 = Unbundle By Name(w205) -> ("Distance (ft)"=w204:dbl, "Center.X"=w184:dbl)
        "Target X Value" <- w184
        n93 = call-poly <vilib>:"NT Read Value.vi"("Name"="Auton Current State") -> ("Numeric"=w193:dbl)  [unwired: 9 in, 1 out]
        n94 = call-poly <vilib>:"NT Write Value.vi"("Numeric"="Defense", "Name"="Auton Defense") -> ()  [unwired: 9 in, 1 out]
        n95 = call "Auton Enum.vi"("Initial State"=w193) -> ("Initial State 2"=→"Auton Current State":T5)  [unwired: 10 in]
        n96 = call-poly <vilib>:"NT Read Value.vi"("Name"="RobotDrive Motors") -> ("Numeric Array"=w222:dbl[])  [unwired: 9 in, 1 out]
        n97 = Build Array(w204, w184) -> (w203:dbl[])
        n98 = call-poly <vilib>:"NT Read Value.vi"("Name"="Gyro Angle") -> ("Numeric"=→"Gyro" →"Gyro Angle":dbl)  [unwired: 9 in, 1 out]
        n99 = call-poly <vilib>:"NT Read Value.vi"("Name"="Shooter at Speed") -> ("Boolean"=→"Shooter at Speed":bool)  [unwired: 9 in, 1 out]
        n100 = Index Array(array=w222, index #1=1, index #4=0) -> (element #1=w238:dbl, element #2=w239:dbl, element #3=w237:dbl, element #4=w242:dbl)  [unwired: 2 in]
        n101 = call-poly <vilib>:"NT Read Value.vi"("Name"="Prep Wheels") -> ("Boolean"=w169:bool)  [unwired: 9 in, 1 out]
        "Shooter Active?" <- w169
        n102 = Bundle("Numeric"=w237, "Numeric"=w238) -> (→"MotorChart R" →"MotorSliders R":cluster{"Numeric":dbl, "Numeric":dbl})  [unwired: 1 in]
        n103 = Bundle("Numeric"=w239, "Numeric"=w242, "Battery V"=w234) -> (→"MotorChart L" →"MotorSliders L":T7)  [unwired: 1 in]
        n104 = call-poly <vilib>:"NT Write Value.vi"("Numeric"="Position", "Name"="Auton Position") -> ()  [unwired: 9 in, 1 out]
        n105 = call-poly <vilib>:"NT Write Value.vi"("Numeric"="Shooter Power", "Name"="Shooter Power") -> ()  [unwired: 9 in, 1 out]
        n106 = property on="Shooter Active?" class="Bool (strict)"("Blinking"=w169) -> ()  [unwired: 2 in, 2 out]
        n107 = call-poly <vilib>:"NT Write Value.vi"("Numeric Array"=w203, "Name"="Target Data") -> ()  [unwired: 9 in, 1 out]
        n108 = call-poly <vilib>:"NT Read Value.vi"("Name"="Shooter Speed") -> ("Numeric"=→"Shooter Speed":dbl)  [unwired: 9 in, 1 out]
        n109 = call-poly <vilib>:"NT Read Value.vi"("Name"="Shooter Setpoint") -> ("Numeric"=→"Shooter Setpoint":dbl)  [unwired: 9 in, 1 out]
        n110 = call-poly <vilib>:"NT Read Value.vi"("Name"="Acquiring?") -> ("Boolean"=→"Acquiring?":bool)  [unwired: 9 in, 1 out]
        n111 = call-poly <vilib>:"NT Write Value.vi"("Boolean"="Gyro Reset", "Name"="Gyro Reset") -> ()  [unwired: 9 in, 1 out]
        n112 = call-poly <vilib>:"NT Read Value.vi"("Name"="Shooter Speed") -> ("Numeric"=→"Shooter Speed (RPS)":dbl)  [unwired: 9 in, 1 out]
        n113 = call-poly <vilib>:"NT Write Value.vi"("Numeric"="Beater Bar Speed", "Name"="Beater Bar Speed") -> ()  [unwired: 9 in, 1 out]
        n114 = call-poly <vilib>:"NT Write Value.vi"("Boolean"="Shooter Control", "Name"="Shooter Control") -> ()  [unwired: 9 in, 1 out]
        n115 = call-poly <vilib>:"NT Write Value.vi"("Numeric"="Shooter Setpoint (RPS)", "Name"="Shooter Setpoint") -> ()  [unwired: 9 in, 1 out]
        n116 = disable-structure shown="Disabled" {
          frame Disabled {
            n117 = call-poly <vilib>:"NT Read Value.vi"("Default Value"=FALSE, "Name"="Rear Camera On?") -> ("Boolean"=→"Rear Camera On?":bool)  [unwired: 8 in, 1 out]
          }
          frame Enabled {
          }
        }
        n118 = disable-structure shown="Disabled" {
          frame Disabled {
            n119 = call-poly <vilib>:"NT Write Value.vi"("Numeric"="Left Compensation", "Name"="Left Compensation") -> ()  [unwired: 9 in, 1 out]
            n120 = call-poly <vilib>:"NT Write Value.vi"("Numeric"="Right Compensation", "Name"="Right Compensation") -> ()  [unwired: 9 in, 1 out]
          }
          frame Enabled {
          }
        }
        n121 = call-poly <vilib>:"NT Write Value.vi"("Numeric"="Top Wheel Speed Multiplier", "Name"="Bottom Wheel Speed Multiplier") -> ()  [unwired: 9 in, 1 out]
        n122 = Index Array(array=w233) -> (element #1=w232:T26, element #2=w227:T26)  [unwired: 2 in]
        n123 = call-poly <vilib>:"NT Read Value.vi"("Name"="Drive Mode") -> ("String"=→"Drive Mode":string)  [unwired: 9 in, 1 out]
        n124 = call-poly <vilib>:"NT Read Value.vi"("Name"="Drive Shift") -> ("String"=→"Drive Shift":string)  [unwired: 9 in, 1 out]
        n125 = call-poly <vilib>:"NT Read Value.vi"("Name"="Hanging Pin") -> ("String"=→"Hanging Pin Status":string)  [unwired: 9 in, 1 out]
        n126 = call "Prepare Joystick Data for Displays.vi"("Joystick Values"=w227) -> ("Buttons"=→"JS2 Buttons":T27, "Z Axis"=→"JS2 Z":dbl, "Cartesian Data"=→"JS2 Graph":cluster{"X axis":dbl, "X axis":dbl}[])  [unwired: 8 in]
        n127 = call "Prepare Joystick Data for Displays.vi"("Joystick Values"=w232) -> ("Buttons"=→"JS1 Buttons":T27, "Z Axis"=→"JS1 Z":dbl, "Cartesian Data"=→"JS1 Graph":cluster{"X axis":dbl, "X axis":dbl}[])  [unwired: 8 in]
        n128 = call-poly <vilib>:"NT Read Value.vi"("Name"="Shooter Speed Top") -> ("Numeric"=→"Shooter Speed Top (RPS)":dbl)  [unwired: 9 in, 1 out]
        n129 = call-poly <vilib>:"NT Write Value.vi"("Boolean"="Auton Shoot", "Name"="Auton Shoot") -> ()  [unwired: 9 in, 1 out]
        n130 = call-poly <vilib>:"NT Write Value.vi"("Numeric"="Shooter Wait (Seconds)", "Name"="Shooter Wait") -> ()  [unwired: 9 in, 1 out]
      }
    }
  }
  n131 = Index Array(array=w51) -> (element=w49:refnum<vi>)  [unwired: 1 in]
  n132 = control-ref of="Test Tree"() -> (w52:refnum<vi>)
  n133 = while {
    tunnel: w49 -> [w255]
    i -> [w258]
    stop <- FALSE stop-if-true
    n134 = Wait (ms)(milliseconds to wait=u32 100) -> ()  [unwired: 1 out]
    n135 = case shown="\"Stop\", Default" "Rec Mode" {
      tunnel: w258 -> [_ _ w273]
      tunnel: [u32 2829099 ("Base Color") u32 11141120 ("Target Color") w262] -> w254
      frame "Stop", Default {
        # "Reset the color, extra updates don't cost much"
      }
      frame "Record" {
      }
      frame "Playback" {
        # "Playback"
        n136 = Quotient & Remainder(x=w273, y=u32 50 ("milliseconds to wait")) -> (x-y*floor(x/y)=w269:u32)  [unwired: 1 out]
        n137 = Divide(x=w269, y=u32 50 ("milliseconds to wait")) -> (x/y=w266:dbl)
        n138 = Multiply(x=6.283185307179586, y=w266) -> (x*y=w271:dbl)
        n139 = Sine(x=w271) -> (sin(x)=w270:dbl)
        n140 = Absolute Value(x=w270) -> (abs(x)=w263:dbl)
        n141 = call "Interpolate RGB Color.vi"("Proportion"=w263, "Target Color"=u32 30976, "Base Color"=u32 2829099) -> ("Result Color"=w262:u32)  [unwired: 8 in]
      }
    }
    n142 = property class="Pane"(reference=w255, "PaneColor"=w254) -> ()  [unwired: 1 in, 2 out]
  }
  n143 = while {
    tunnel: w55 -> [w285]
    shift-right: [w284] -> _
    shift-left: w53 -> [w283]
    tunnel: [w282] -> _
    tunnel: w52 -> [w281]
    tunnel: w48 -> [w280]
    tunnel: w47 -> [w279]
    tunnel: w46 -> [_]
    tunnel: w42 -> [w278]
    tunnel: w5 -> [w277]
    tunnel: w3 -> [w276]
    shift-right: [w275] -> _
    shift-left: _ -> [w274]
    i -> [w282]
    stop <- FALSE stop-if-true
    n144 = event shown="[18] \"Rec Mode\": Value Change" {
      selector: w279 -> [_ _ _ _ _ _ _ _ _ _ _ _ _ _ _ _ _ _ _ _ _ _ _ _]
      dyn-events: [_ _ _ _ _ _ _ _ _ _ _ _ _ _ _ _ _ _ w594 _ _ _ _ _] -> _
      timeout: u32 60 ("milliseconds to wait") -> [_ _ _ _ _ _ _ _ _ _ _ _ _ _ _ _ _ _ _ _ _ _ _ _]
      tunnel: w281 -> [w298 _ _ _ _ _ _ _ _ _ _ _ _ _ _ _ _ _ _ _ _ _ _ _]
      tunnel: "Test Tree" -> [_ _ _ _ _ _ _ _ _ _ _ _ _ w557 w566 w569 w574 w583 _ _ _ _ _ _]
      tunnel: w285 -> [_ w336 _ _ _ _ _ _ _ _ _ w519 w550 _ _ _ _ _ _ _ _ _ _ _]
      tunnel: [w295 w335 w439 w445 w455 w459 w465 w477 w485 w491 w504 w518 w543 w556 w564 w568 w573 w582 w596 w612 w614 w622 w633 w638] -> w284
      tunnel: w283 -> [w295 w335 w439 w445 w455 w459 w465 w477 w485 w491 w504 w517 w543 w556 w564 w568 w573 w582 w596 w612 w614 w622 w633 w638]
      tunnel: w280 -> [_ _ _ _ _ _ _ _ _ _ _ _ _ _ _ _ _ _ w597 _ w617 _ _ _]
      tunnel: w278 -> [_ _ _ _ _ _ _ _ _ _ _ _ _ _ _ _ _ _ w592 _ _ _ _ _]
      tunnel: w277 -> [_ _ _ _ _ _ _ _ _ _ _ _ _ _ _ _ _ _ w588 _ _ _ _ _]
      tunnel: w276 -> [w290 _ _ _ _ _ w463 _ _ _ _ _ _ _ _ _ _ _ _ _ _ _ _ _]
      tunnel: [w289 w334 w438 w444 w454 w460 w461 w471 w482 w490 w503 w516 w542 w555 w563 w567 w572 w581 w587 w610 w613 w618 w626 w639] -> w275
      tunnel: w274 -> [w289 w334 w438 w444 w454 w460 w461 _ _ w490 w503 w516 w542 w555 w563 w567 w572 w581 w587 w610 w613 w618 w626 w639]
      event Timeout {
        n145 = event-data() -> ()  [unwired: 1 in, 1 out]
        n146 = local read "Mode"() -> (w292:T10)
        n147 = call <vilib>:"NT Read String.vi"("Name"="/TestMode/TestName") -> ("String"=w301:string)  [unwired: 9 in, 1 out]
        n148 = case shown="\"Diagnostics\", Default" "Dashboard Tab" {
          tunnel: w298 -> [_ w312 _ _]
          tunnel: "/TestMode/Automatic/" ("Name Pattern") -> [_ w311 _ _]
          tunnel: T28 [{"Operation"=enum."Clear", "Color Box"=14013909}, {"Operation"=enum."Clear", "Color Box"=14013909}, {"Operation"=enum."Clear", "Color Box"=14013909}, {"Operation"=enum."Clear", "Color Box"=14013909}, {"Operation"=enum."Update", "Color Box"=14013909}, {"Operation"=enum."Update", "Color Box"=16777215}, {"Operation"=enum."Clear", "Color Box"=14013909}, {"Operation"=enum."Clear", "Color Box"=14013909}, {"Operation"=enum."Clear", "Color Box"=14013909}] -> [_ w304 _ w321]
          tunnel: w292 -> [_ w303 _ w320]
          tunnel: u32[] [15790320, 15790320, 15790320, 15790320, 16777215, 16777215, 15790320, 15790320, 15790320] -> [_ _ _ w326]
          tunnel: w290 -> [_ _ _ w314]
          frame "Diagnostics", Default {
          }
          frame "Test" {
            w310 = -2 ("Active Item:Row Number")
            n149 = Index Array(array=w304, index=w303) -> (element=w305:T32)
            n150 = Unbundle(w305) -> ("Operation"=w306:enum16{"Update", "Clear"}, "Color Box"=w307:u32)
            n151 = call <vilib>:"NT Read and Format Entries as Tree.vi"("Operation"=w306, "Name Pattern"=w311, "Tree Refnum"=w312) -> ()  [unwired: 7 in, 2 out]
            n152 = property on="Test Tree" class="Tree (strict)"("Active Item Row Number"=w310, "ActiveColNum"=w310, "CellBG"=w307, "Active Item Row Number"=-1 ("Active Item:Row Number"), "CellBG"=u32 5789784 ("Color Box")) -> ()  [unwired: 2 in, 2 out]
          }
          frame "Variables" {
            n153 = control-ref of="Tree"() -> (w313:refnum<vi>)
            n154 = call <vilib>:"NT Read and Format Entries as Tree.vi"("Tree Refnum"=w313) -> ()  [unwired: 9 in, 2 out]
          }
          frame "Commands" {
            w322 = u32 5789784 ("Color Box")
            w323 = T33 {"Row"=-1, "Column"=-2} ("Active Cell:Active Cell")
            w325 = T33 {"Row"=-2, "Column"=-2} ("Active Cell:Active Cell")
            n155 = Index Array(array=w326, index=w320) -> (element=w324:u32)
            n156 = Index Array(array=w321, index=w320) -> (element=w319:T32)
            n157 = Unbundle(w319) -> ("Operation"=w318:enum16{"Update", "Clear"})  [unwired: 1 out]
            n158 = local read "Command Selection"() -> (w317:i32)
            n159 = property on="Command Selection" class="MCListbox (strict)"("ActiveCell"=w325, "CellBG"=w324, "ActiveCell"=w323, "CellBG"=w322) -> ()  [unwired: 2 in, 2 out]
            n160 = call <vilib>:"WPI_DashboardUpdate RPC Info.vi"("Operation"=w318) -> ("update"=w316:bool, "commands"=w315:string[][])  [unwired: 9 in]
            n161 = property on="Command Selection" class="MCListbox (strict)"("ItemNames"=w315) -> ()  [unwired: 2 in, 2 out]
            n162 = property on="Command Params" class="Tbl (strict)"("Active Cell"=w325, "Cell BG Color"=w324, "Active Cell"=w323, "Cell BG Color"=w322) -> ()  [unwired: 2 in, 2 out]
            n163 = call <vilib>:"WPI_DashboardUpdate Command Params.vi"("Update"=w316, "NewVal"=w317, "Commands"=w315, "Param Tbl"=w314) -> ()  [unwired: 7 in, 1 out]
          }
        }
        n164 = case shown="\"\"" w301 {
          tunnel: "/TestMode/TestProgress" ("Name") -> [w328 _]
          tunnel: "/TestMode/TestProgressText" ("Name") -> [w327 _]
          frame Default {
            n165 = call <vilib>:"NT Read Number.vi"("Name"=w328) -> ("Numeric"=w329:dbl)  [unwired: 9 in, 1 out]
            n166 = call <vilib>:"NT Read String.vi"("Name"=w327) -> ("String"=w330:string)  [unwired: 9 in, 1 out]
            n167 = Bundle("Numeric"=w329, "String"=w330) -> (→"Progress":cluster{"Numeric":dbl, "String":string})  [unwired: 1 in]
          }
          frame "" {
            n168 = property on="Progress" class="Clust (strict)"("Visible"=FALSE) -> ()  [unwired: 2 in, 2 out]
            n169 = local write "Test Name"(u16 0) -> ()
          }
        }
        n170 = call <vilib>:"Connextion Info.vi"() -> ("Connected"=→"NT Connection":bool)  [unwired: 10 in, 1 out]
      }
      event "Test Tree": Value Change {
        # "Show appropriate\ncontrols"
        n171 = event-data() -> ("CtlRef"=w339:refnum<vi>, "NewVal"=w337:string)  [unwired: 1 in]
        n172 = call <vilib>:"WPI_UtilitiesGetTreeIOName.vi"("NewVal"=w337, "TreeControl in"=w339) -> ("I/O Name"=w340:string)  [unwired: 9 in]
        n173 = case shown="\"Analog Out\", \"Motor\", \"PWM\"" w340 {
          selector: w340 -> [_ w347 _ w369 w378 _]
          tunnel: w337 -> [_ _ w366 w368 _ w385]
          tunnel: w336 -> [_ _ _ _ _ w384]
          frame Default {
            w342 = FALSE ("Visible")
            w341 = FALSE ("Visible")
            n174 = property on="Motor" class="Clust (strict)"("Visible"=w341) -> ()  [unwired: 2 in, 2 out]
            n175 = property on="Test Ring" class="Ring (strict)"("Visible"=w341) -> ()  [unwired: 2 in, 2 out]
            n176 = property on="Rev/Fwd" class="Clust (strict)"("Visible"=w342) -> ()  [unwired: 2 in, 2 out]
            n177 = property on="On/Off" class="Bool (strict)"("Visible"=w342) -> ()  [unwired: 2 in, 2 out]
            n178 = property on="Test Slider" class="Slide (strict)"("Visible"=w342) -> ()  [unwired: 2 in, 2 out]
          }
          frame "Analog Out", "Motor", "PWM" {
            w348 = FALSE ("Visible")
            n179 = case shown="\"Analog Out\"" w347 {
              tunnel: [1.0 ("Value") -1.0 ("Value") 0.0 ("Value")] -> w346
              tunnel: [255.0 ("Value") 1.0 ("Value") 5.0 ("Value")] -> w345
              tunnel: [128.0 ("Value") 0.0 ("Value") 0.0 ("Value")] -> w344
              tunnel: [64.0 ("Value") 0.5 ("Value") 1.0 ("Value")] -> w343
              frame "PWM" {
              }
              frame "Motor", Default {
              }
              frame "Analog Out" {
              }
            }
            n180 = property on="Motor" class="Clust (strict)"("Visible"=TRUE) -> ()  [unwired: 2 in, 2 out]
            n181 = property on="Value" class="Slide (strict)"("Value"=w344, "Scale.Minimum"=w346, "Scale.Maximum"=w345, "Scale.Increment"=w343) -> ()  [unwired: 2 in, 2 out]
            n182 = property on="On/Off" class="Bool (strict)"("Visible"=w348) -> ()  [unwired: 2 in, 2 out]
            n183 = property on="Test Slider" class="Slide (strict)"("Visible"=w348) -> ()  [unwired: 2 in, 2 out]
            n184 = property on="Test Ring" class="Ring (strict)"("Visible"=w348) -> ()  [unwired: 2 in, 2 out]
            n185 = property on="Rev/Fwd" class="Clust (strict)"("Visible"=w348) -> ()  [unwired: 2 in, 2 out]
          }
          frame "Servo" {
            w364 = FALSE ("Visible")
            n186 = call <vilib>:"NT Read Number.vi"("Name"=w366) -> ("Numeric"=w365:dbl)  [unwired: 9 in, 1 out]
            n187 = property on="Test Slider" class="Slide (strict)"("Visible"=TRUE, "Scale.Maximum"=170.0 ("Scale.Range:Maximum")) -> ()  [unwired: 2 in, 2 out]
            n188 = local write "Test Slider"(w365) -> ()
            n189 = property on="Motor" class="Clust (strict)"("Visible"=w364) -> ()  [unwired: 2 in, 2 out]
            n190 = property on="Rev/Fwd" class="Clust (strict)"("Visible"=w364) -> ()  [unwired: 2 in, 2 out]
            n191 = property on="On/Off" class="Bool (strict)"("Visible"=w364) -> ()  [unwired: 2 in, 2 out]
            n192 = property on="Test Ring" class="Ring (strict)"("Visible"=w364) -> ()  [unwired: 2 in, 2 out]
          }
          frame "Relay", "Solenoid" {
            w367 = FALSE ("Visible")
            n193 = property on="Motor" class="Clust (strict)"("Visible"=w367) -> ()  [unwired: 2 in, 2 out]
            n194 = property on="Test Slider" class="Slide (strict)"("Visible"=w367) -> ()  [unwired: 2 in, 2 out]
            n195 = Search and Replace String(input string=w368, search string="/Value  **", replace string="/Direction") -> (result string=w374:string)  [unwired: 5 in, 3 out]
            n196 = property on="Test Ring" class="Ring (strict)"("Visible"=w367) -> ()  [unwired: 2 in, 2 out]
            n197 = call <vilib>:"NT Read String.vi"("Name"=w374) -> ("String"=w372:string)  [unwired: 9 in, 1 out]
            n198 = Equal?(x="Both directions", y=w372) -> (x = y?=w370:bool)
            n199 = Not(x=w370) -> (.not. x?=w371:bool)
            n200 = property on="Rev/Fwd" class="Clust (strict)"("Visible"=w370) -> ()  [unwired: 2 in, 2 out]
            n201 = property on="On/Off" class="Bool (strict)"("Visible"=w371, "Caption.Text"=w369) -> ()  [unwired: 2 in, 2 out]
          }
          frame "Compressor", "Digital Out" {
            w377 = FALSE ("Visible")
            # "Get direction and finish"
            n202 = property on="Motor" class="Clust (strict)"("Visible"=w377) -> ()  [unwired: 2 in, 2 out]
            n203 = property on="Test Slider" class="Slide (strict)"("Visible"=w377) -> ()  [unwired: 2 in, 2 out]
            n204 = property on="Test Ring" class="Ring (strict)"("Visible"=w377) -> ()  [unwired: 2 in, 2 out]
            n205 = property on="On/Off" class="Bool (strict)"("Visible"=TRUE, "Caption.Text"=w378) -> ()  [unwired: 2 in, 2 out]
            n206 = property on="Rev/Fwd" class="Clust (strict)"("Visible"=FALSE) -> ()  [unwired: 2 in, 2 out]
          }
          frame "Camera" {
            n207 = call <vilib>:"Get Last Path Segment.vi"("String in"=w385) -> ("String out"=w386:string)  [unwired: 10 in]
            n208 = property on="On/Off" class="Bool (strict)"("Visible"=FALSE) -> ()  [unwired: 2 in, 2 out]
            n209 = property on="Motor" class="Clust (strict)"("Visible"=FALSE) -> ()  [unwired: 2 in, 2 out]
            n210 = property on="Rev/Fwd" class="Clust (strict)"("Visible"=FALSE) -> ()  [unwired: 2 in, 2 out]
            n211 = case shown="\"White Balance  **\"" w386 {
              tunnel: w385 -> [w392 w401 w410 w419 w428 _ w434]
              tunnel: w384 -> [w390 w398 w407 w416 w425 _ _]
              frame "Size  **" {
                n212 = Index Array(array=w390) -> (element=w389:cluster{string[]})  [unwired: 1 in]
                n213 = call <vilib>:"NT Read String.vi"("Name"=w392) -> ("String"=w391:string)  [unwired: 9 in, 1 out]
                n214 = Unbundle(w389) -> (w387:string[])
                n215 = Match First String(2:w387, 3:w391) -> (0:w388:i32)  [unwired: 1 out]
                n216 = property on="Test Ring" class="Ring (strict)"("Value"=w388, "Strings []"=w387) -> ()  [unwired: 2 in, 2 out]
                n217 = property on="Test Ring" class="Ring (strict)"("Visible"=TRUE) -> ()  [unwired: 2 in, 2 out]
                n218 = property on="Test Slider" class="Slide (strict)"("Visible"=FALSE) -> ()  [unwired: 2 in, 2 out]
              }
              frame "White Balance  **" {
                n219 = Index Array(array=w398, index=1) -> (element=w399:cluster{string[]})
                n220 = call <vilib>:"NT Read String.vi"("Name"=w401) -> ("String"=w400:string)  [unwired: 9 in, 1 out]
                n221 = Unbundle(w399) -> (w396:string[])
                n222 = Match First String(2:w396, 3:w400) -> (0:w395:i32)  [unwired: 1 out]
                n223 = property on="Test Ring" class="Ring (strict)"("Value"=w395, "Strings []"=w396) -> ()  [unwired: 2 in, 2 out]
                n224 = property on="Test Ring" class="Ring (strict)"("Visible"=TRUE) -> ()  [unwired: 2 in, 2 out]
                n225 = property on="Test Slider" class="Slide (strict)"("Visible"=FALSE) -> ()  [unwired: 2 in, 2 out]
              }
              frame "Exposure  **" {
                n226 = Index Array(array=w407, index=2) -> (element=w408:cluster{string[]})
                n227 = call <vilib>:"NT Read String.vi"("Name"=w410) -> ("String"=w409:string)  [unwired: 9 in, 1 out]
                n228 = Unbundle(w408) -> (w404:string[])
                n229 = Match First String(2:w404, 3:w409) -> (0:w405:i32)  [unwired: 1 out]
                n230 = property on="Test Ring" class="Ring (strict)"("Value"=w405, "Strings []"=w404) -> ()  [unwired: 2 in, 2 out]
                n231 = property on="Test Ring" class="Ring (strict)"("Visible"=TRUE) -> ()  [unwired: 2 in, 2 out]
                n232 = property on="Test Slider" class="Slide (strict)"("Visible"=FALSE) -> ()  [unwired: 2 in, 2 out]
              }
              frame "Exposure Priority  **" {
                n233 = Index Array(array=w416, index=3) -> (element=w417:cluster{string[]})
                n234 = call <vilib>:"NT Read String.vi"("Name"=w419) -> ("String"=w418:string)  [unwired: 9 in, 1 out]
                n235 = Unbundle(w417) -> (w413:string[])
                n236 = Match First String(2:w413, 3:w418) -> (0:w414:i32)  [unwired: 1 out]
                n237 = property on="Test Ring" class="Ring (strict)"("Value"=w414, "Strings []"=w413) -> ()  [unwired: 2 in, 2 out]
                n238 = property on="Test Ring" class="Ring (strict)"("Visible"=TRUE) -> ()  [unwired: 2 in, 2 out]
                n239 = property on="Test Slider" class="Slide (strict)"("Visible"=FALSE) -> ()  [unwired: 2 in, 2 out]
              }
              frame "Color Enable  **" {
                n240 = Index Array(array=w425, index=4) -> (element=w426:cluster{string[]})
                n241 = call <vilib>:"NT Read String.vi"("Name"=w428) -> ("String"=w427:string)  [unwired: 9 in, 1 out]
                n242 = Unbundle(w426) -> (w422:string[])
                n243 = Match First String(2:w422, 3:w427) -> (0:w423:i32)  [unwired: 1 out]
                n244 = property on="Test Ring" class="Ring (strict)"("Value"=w423, "Strings []"=w422) -> ()  [unwired: 2 in, 2 out]
                n245 = property on="Test Ring" class="Ring (strict)"("Visible"=TRUE) -> ()  [unwired: 2 in, 2 out]
                n246 = property on="Test Slider" class="Slide (strict)"("Visible"=FALSE) -> ()  [unwired: 2 in, 2 out]
              }
              frame Default {
                n247 = property on="Test Ring" class="Ring (strict)"("Visible"=FALSE) -> ()  [unwired: 2 in, 2 out]
                n248 = property on="Test Slider" class="Slide (strict)"("Visible"=FALSE) -> ()  [unwired: 2 in, 2 out]
              }
              frame "Brightness  **", "Color Level  **", "Compression  **", "FPS  **", "Sharpness  **" {
                n249 = call <vilib>:"NT Read Number.vi"("Name"=w434) -> ("Numeric"=w433:dbl)  [unwired: 9 in, 1 out]
                n250 = local write "Test Slider"(w433) -> ()
                n251 = property on="Test Slider" class="Slide (strict)"("Visible"=TRUE, "Scale.Maximum"=100.0 ("Scale.Range:Maximum")) -> ()  [unwired: 2 in, 2 out]
                n252 = property on="Test Ring" class="Ring (strict)"("Visible"=FALSE) -> ()  [unwired: 2 in, 2 out]
              }
            }
          }
        }
        n253 = property on="Progress" class="Clust (strict)"("Visible"=FALSE) -> ()  [unwired: 2 in, 2 out]
      }
      event "Test Name": Mouse Enter {
        # "Populate the ring with the list of tests"
        n254 = event-data() -> ()  [unwired: 1 in, 1 out]
        n255 = call <vilib>:"NT Read String Array.vi"("Name"="/TestMode/TestList") -> ("String Array"=w443:string[])  [unwired: 9 in, 1 out]
        n256 = Build Array (concatenate)("Select the test to run...", w443) -> (w442:string[])
        n257 = property on="Test Name" class="Ring (strict)"("Strings []"=w442) -> ()  [unwired: 2 in, 2 out]
      }
      event "Test Name": Value Change {
        w446 = FALSE ("Visible")
        # "Tell the robot the test name to run"
        n258 = event-data() -> ("NewVal"=w450:u16)  [unwired: 1 in]
        n259 = property on="Test Name" class="Ring (strict)"() -> ("Strings []"=w451:string[])  [unwired: 2 in, 2 out]
        n260 = local write "Progress"(T12 {"Test Progress"=0, "Test Progress Text"=""} ("Progress")) -> ()
        n261 = Index Array(array=w451, index=w450) -> (element=w449:string)
        n262 = call <vilib>:"NT Write String.vi"("String"=w449, "Name"="/TestMode/TestName") -> ()  [unwired: 9 in, 1 out]
        n263 = property on="Progress" class="Clust (strict)"("Visible"=TRUE) -> ()  [unwired: 2 in, 2 out]
        n264 = property on="Motor" class="Clust (strict)"("Visible"=w446) -> ()  [unwired: 2 in, 2 out]
        n265 = property on="Test Slider" class="Slide (strict)"("Visible"=w446) -> ()  [unwired: 2 in, 2 out]
        n266 = property on="On/Off" class="Bool (strict)"("Visible"=w446) -> ()  [unwired: 2 in, 2 out]
        n267 = property on="Rev/Fwd" class="Clust (strict)"("Visible"=w446) -> ()  [unwired: 2 in, 2 out]
        n268 = property on="Test Ring" class="Ring (strict)"("Visible"=w446) -> ()  [unwired: 2 in, 2 out]
      }
      event "Select Auto": Mouse Enter {
        # "Populate the combo box with the list of autonomous options"
        n269 = event-data() -> ()  [unwired: 1 in, 1 out]
        n270 = call <vilib>:"NT Read String Array.vi"("Name"="Auto List") -> ("String Array"=w453:string[])  [unwired: 9 in, 1 out]
        n271 = property on="Select Auto" class="CmbBox"("Strings[]"=w453) -> ()  [unwired: 2 in, 2 out]
      }
      event "Select Auto": Value Change {
        # "User modified the Auto Selection. Write to NT variable so robot knows."
        n272 = event-data() -> ("NewVal"=w457:string)  [unwired: 1 in]
        n273 = call <vilib>:"NT Write String.vi"("String"=w457, "Name"="Auto Selector") -> ()  [unwired: 9 in, 1 out]
      }
      event "Command Selection": Value Change {
        # "Get the params and show in table"
        n274 = event-data() -> ("NewVal"=w464:i32)  [unwired: 1 in]
        n275 = property on="Command Selection" class="MCListbox (strict)"() -> ("ItemNames"=w462:string[][])  [unwired: 2 in, 2 out]
        n276 = call <vilib>:"WPI_DashboardUpdate Command Params.vi"("NewVal"=w464, "Commands"=w462, "Param Tbl"=w463) -> ()  [unwired: 8 in, 1 out]
      }
      event "Execute Command": Value Change {
        # "Started one, Unique ID holds\nresponse"
        n277 = event-data() -> ()  [unwired: 1 in, 1 out]
        n278 = property on="Command Selection" class="MCListbox (strict)"() -> ("ItemNames"=w476:string[][])  [unwired: 2 in, 2 out]
        n279 = Index Array(array=w476, index (row)="Command Selection", index (col)=0) -> (element=w474:string)
        n280 = call <vilib>:"Invoke Commands.vi"("Command Params"="Command Params", "Function Name"=w474) -> ("Params"=w470:u8, "Started"=w469:bool)  [unwired: 7 in, 1 out]
        n281 = Array Subset(array="Command Params", length (row)=w470) -> (w471:string[][])  [unwired: 3 in]
        n282 = Select(t="Executing" ("Cmd Status"), s=w469, f="" ("Cmd Status")) -> (s? t:f=→"Cmd Status":string)
      }
      event "Command Selection": Double Click {
        n283 = event-data() -> ("Row"=w486:i32)  [unwired: 1 in]
        n284 = property on="Command Selection" class="MCListbox (strict)"() -> ("ItemNames"=w489:string[][])  [unwired: 2 in, 2 out]
        n285 = local read "Command Params"() -> (w484:string[][])
        n286 = Index Array(array=w489, index (row)=w486, index (col)=0) -> (element=w487:string)
        n287 = call <vilib>:"Invoke Commands.vi"("Command Params"=w484, "Function Name"=w487) -> ("Params"=w483:u8, "Started"=w478:bool)  [unwired: 7 in, 1 out]
        n288 = Array Subset(array=w484, length (row)=w483) -> (w482:string[][])  [unwired: 3 in]
        n289 = Select(t="Executing" ("Cmd Status"), s=w478, f="" ("Cmd Status")) -> (s? t:f=w479:string)
        n290 = local write "Cmd Status"(w479) -> ()
      }
      event "CheckList": Double Click {
        # "Shift clears all"
        # "Update symbols on the listbox"
        n291 = event-data() -> ("PlatMods.Shift"=w492:bool, "Row"=w494:i32)  [unwired: 1 in]
        n292 = case shown="True" w492 {
          tunnel: w494 -> [w498 _]
          tunnel: 1 -> [w497 _]
          frame False {
            n293 = property on="CheckList" class="LstBox (strict)"() -> ("Item Symbols"=w496:i32[])  [unwired: 2 in, 2 out]
            n294 = Replace Array Subset(array=w496, new element=w497, index=w498) -> (w495:i32[])
            n295 = property on="CheckList" class="LstBox (strict)"("Item Symbols"=w495) -> ()  [unwired: 2 in, 2 out]
          }
          frame True {
            w499 = 0 ("Top Row")
            n296 = property on="CheckList" class="LstBox (strict)"() -> ("Number of Rows"=w501:u32)  [unwired: 2 in, 2 out]
            n297 = Initialize Array(0, w501) -> (w500:i32[])
            n298 = property on="CheckList" class="LstBox (strict)"("Top Row"=w499, "Value"=w499, "Item Symbols"=w500) -> ()  [unwired: 2 in, 2 out]
          }
        }
      }
      event "CheckList": Key Down {
        # "Update symbols on the listbox\nLeft and right keys check and uncheck"
        n299 = event-data() -> ("VKey"=w506:T29)  [unwired: 1 in]
        n300 = case shown="\"Left\", \"Right\"" w506 {
          selector: w506 -> [w511 _]
          tunnel: eventvkey."Left" ("VKey") -> [w509 _]
          frame "Left", "Right" {
            n301 = Equal?(x=w509, y=w511) -> (x = y?=w510:bool)
            n302 = Select(t=0, s=w510, f=1) -> (s? t:f=w512:i32)
            n303 = property on="CheckList" class="LstBox (strict)"() -> ("Item Symbols"=w515:i32[])  [unwired: 2 in, 2 out]
            n304 = Replace Array Subset(array=w515, new element=w512, index="CheckList") -> (w514:i32[])
            n305 = property on="CheckList" class="LstBox (strict)"("Item Symbols"=w514) -> ()  [unwired: 2 in, 2 out]
          }
          frame Default {
          }
        }
      }
      event "DB Camera Config": Value Change {
        # "Show or hide the cluster of controls, store in ini file"
        n306 = event-data() -> ("NewVal"=w520:bool)  [unwired: 1 in]
        n307 = case shown="False" w520 {
          tunnel: w519 -> [w529 _]
          tunnel: [w522 w540] -> w518
          tunnel: w517 -> [w521 w540]
          frame False {
            w536 = "Camera"
            w539 = FALSE ("Visible")
            n308 = local read "Camera Settings"() -> (w528:T6)
            n309 = Index Array(array=w529) -> (element=w532:cluster{string[]})  [unwired: 1 in]
            n310 = Unbundle(w528) -> ("Frame Rate"=w527:i32, "Compression"=w526:i32, "Size"=w530:u16)
            n311 = Unbundle(w532) -> (w531:string[])
            n312 = Index Array(array=w531, index=w530) -> (element=w525:string)
            n313 = call-poly <vilib>:"Write Key.vi"("section"=w536, "value"=w525, "key"="Size", "refnum"=w521) -> ("refnum out"=w538:T18)  [unwired: 2 in, 5 out]
            n314 = call-poly <vilib>:"Write Key.vi"("section"=w536, "value"=w527, "key"="FrameRate", "refnum"=w538) -> ("refnum out"=w537:T18)  [unwired: 1 in, 6 out]
            n315 = property on="Camera Settings" class="Clust (strict)"("Visible"=w539) -> ()  [unwired: 2 in, 2 out]
            n316 = local write "DB Camera Config"(w539) -> ()
            n317 = call-poly <vilib>:"Write Key.vi"("section"=w536, "value"=w526, "key"="Compression", "refnum"=w537) -> ("refnum out"=w523:T18)  [unwired: 1 in, 6 out]
            n318 = call <vilib>:"Close Config Data.vi"("refnum"=w523) -> ("file path"=w524:path)  [unwired: 2 in, 8 out]
            n319 = call <vilib>:"Open Config Data.vi"("configuration file path"=w524) -> ("refnum"=w522:T18)  [unwired: 8 in, 2 out]
          }
          frame True {
            n320 = property on="Camera Settings" class="Clust (strict)"("Visible"=TRUE) -> ()  [unwired: 2 in, 2 out]
          }
        }
      }
      event "Camera Settings": Value Change {
        # "Update summary string when any elements of DB camera change"
        n321 = event-data() -> ("NewVal"=w554:T6)  [unwired: 1 in]
        n322 = Index Array(array=w550) -> (element=w549:cluster{string[]})  [unwired: 1 in]
        n323 = Unbundle(w554) -> ("Frame Rate"=w545:i32, "Compression"=w544:i32, "Size"=w547:u16)
        n324 = Unbundle(w549) -> (w548:string[])
        n325 = Index Array(array=w548, index=w547) -> (element=w546:string)
        n326 = Format Into String(format string="%s   %dfps   %d%%", w546, w545, w544) -> (resulting string=w551:string)  [unwired: 2 in, 1 out]
        n327 = Build Array(w551) -> (w552:string[])
        n328 = property on="DB Camera Config" class="Bool (strict)"("Strings [4]"=w552) -> ()  [unwired: 2 in, 2 out]
      }
      event "Motor.Enable": Value Change {
        # "When the test mode otor enable helper is set, update that\ntree row item's value"
        n329 = event-data() -> ("NewVal"=w561:bool)  [unwired: 1 in]
        n330 = Unbundle("Motor") -> ("Value"=w560:dbl)  [unwired: 1 out]
        n331 = Select(t=w560, s=w561, f=0.0) -> (s? t:f=w558:dbl)
        n332 = call <vilib>:"NT Write Number.vi"("Numeric"=w558, "Name"=w557) -> ()  [unwired: 9 in, 1 out]
      }
      event "Test Slider": Value Change {
        # "When the test mode slider helper is set, update that\ntree row item's value"
        n333 = event-data() -> ("NewVal"=w565:dbl)  [unwired: 1 in]
        n334 = call <vilib>:"NT Write Number.vi"("Numeric"=w565, "Name"=w566) -> ()  [unwired: 9 in, 1 out]
      }
      event "On/Off": Value Change {
        # "When the test mode on/off helper value is set, update that\ntree row item's value"
        n335 = event-data() -> ("NewVal"=w571:bool)  [unwired: 1 in]
        n336 = Boolean To (0,1)(Boolean=w571) -> (0, 1=w570:i16)
        n337 = call <vilib>:"NT Write Number.vi"("Numeric"=w570, "Name"=w569) -> ()  [unwired: 9 in, 1 out]
      }
      event "Rev/Fwd": Value Change {
        # "When the test mode helper value for relays is set, update that\ntree row item's value"
        n338 = event-data() -> ("NewVal.Forward"=w580:bool, "NewVal.Reverse"=w579:bool)  [unwired: 1 in]
        n339 = Boolean To (0,1)(Boolean=w580) -> (0, 1=w576:i16)
        n340 = Boolean To (0,1)(Boolean=w579) -> (0, 1=w578:i16)
        n341 = Negate(x=w578) -> (-x=w577:i16)
        n342 = Add(x=w576, y=w577) -> (x+y=w575:i16)
        n343 = call <vilib>:"NT Write Number.vi"("Numeric"=w575, "Name"=w574) -> ()  [unwired: 9 in, 1 out]
      }
      event "Test Ring": Value Change {
        # "When a test mode helper value is selected from the ring,\nset the tree item's variable to the string value"
        n344 = event-data() -> ("NewVal"=w585:u16)  [unwired: 1 in]
        n345 = property on="Test Ring" class="Ring (strict)"() -> ("Strings []"=w586:string[])  [unwired: 2 in, 2 out]
        n346 = Index Array(array=w586, index=w585) -> (element=w584:string)
        n347 = call <vilib>:"NT Write String.vi"("String"=w584, "Name"=w583) -> ()  [unwired: 9 in, 1 out]
      }
      event "Rec Mode": Value Change {
        # "Update globals for recording mode and path to read log from.\nClear when logging and let NetworkTables set path for vision to\nuse."
        n348 = event-data() -> ("NewVal"=w598:enum32{"Stop", "Record", "Playback"})  [unwired: 1 in]
        n349 = global write "WPI_DashboardLogging Global.vi" "Logging Filename"(path "") -> ()
        n350 = global write "WPI_DashboardLogging Global.vi" "Recording"(w598) -> ()
        n351 = case shown="\"Playback\"" w598 {
          tunnel: w597 -> [_ w600 w609]
          tunnel: [_ _ w608] -> w594
          tunnel: [_ _ w607] -> _
          tunnel: w592 -> [_ _ w605]
          tunnel: cluster{i32, i32} {-250, 170} -> [_ _ w604]
          tunnel: [_ _ T30 {"Image Size"=TRUE, "Image Type"=TRUE, "Pixel Value"=TRUE, "ROI Information"=TRUE, "Zoom Factor"=FALSE} ("Image Information Shown:All Elements")] -> w590
          tunnel: [_ _ TRUE ("Zoom Factor")] -> w589
          tunnel: w588 -> [_ _ w601]
          frame Default {
          }
          frame "Stop", "Record" {
            # "Place Window too"
            n352 = invoke class="VI" method="FP.Close"(reference=w600) -> (reference out=w599:refnum<vi>)  [unwired: 2 in, 2 out]
            n353 = invoke class="VI" method="Abort VI"(reference=w599) -> ()  [unwired: 2 in, 3 out]
          }
          frame "Playback" {
            n354 = call "Open Playback Panel.vi"("Offset"=w604, "DB VI Ref"=w605, "Playback in"=w609) -> ("Playback out"=w606:refnum<vi>)  [unwired: 8 in]
            n355 = register-events(w606, w601) -> (reference out=w608:refnum<event-registration>, error out=w607:errorcluster)  [unwired: 2 in]
          }
        }
        n356 = property on="Unmasked Image" class="ImageControl"("Image Information Shown"=w590, "Image Information Visible"=w589) -> ()  [unwired: 2 in, 2 out]
        n357 = call <vilib>:"WPI_DashboardNT Log FieldName Cache.vi"("Operation"=enum16{"Lookup/Add", "Index", "Clear"}."Clear") -> ()  [unwired: 8 in, 3 out]
      }
      event Panel Close {
        w611 = enum32{"Stop", "Record", "Playback"}."Stop" ("Rec Mode")
        # "Playback window has been closed, abort"
        n358 = event-data() -> ()  [unwired: 1 in, 4 out]
        n359 = local write "Rec Mode"(w611) -> ()
        n360 = global write "WPI_DashboardLogging Global.vi" "Recording"(w611) -> ()
      }
      event Panel Close {
        # "Abort playback window and ourself"
        n361 = event-data() -> ()  [unwired: 1 in, 4 out]
        n362 = invoke class="VI" method="FP.Close"(reference=w617) -> (reference out=w616:refnum<vi>)  [unwired: 2 in, 2 out]
        n363 = invoke class="VI" method="Abort VI"(reference=w616) -> (error out=w615:errorcluster)  [unwired: 2 in, 2 out]
        n364 = invoke class="VI" method="Abort VI"(error in=w615) -> ()  [unwired: 2 in, 3 out]
      }
      event User Event {
        n365 = event-data() -> ("IDs"=w625:cluster{"RPC field ID":u16, "Unique ID":u16}, "String"=w624:string)  [unwired: 1 in]
        n366 = Bundle("IDs"=w625, "String"=w624) -> (w623:T14)  [unwired: 1 in]
        n367 = call <vilib>:"Retrieve RPC Response.vi"("RPC Response"=w623) -> ("Output"=w620:string[][])  [unwired: 10 in]
        n368 = Build Array (concatenate)(w618, w620) -> (w619:string[][])
        n369 = local write "Command Params"(w619) -> ()
        n370 = local write "Cmd Status"("" ("Cmd Status")) -> ()
      }
      event "Vision": Value Change {
        # "Enable/Disable Compression slider.\nHW USB is hard-coded into the camera"
        n371 = event-data() -> ("NewVal"=w632:u16)  [unwired: 1 in]
        n372 = Equal?(x=w632, y=u32 2 ("milliseconds to wait")) -> (x = y?=w630:bool)
        n373 = Select(t=T31."Disabled and Grayed Out" ("Disabled"), s=w630, f=T31."Enabled" ("Disabled")) -> (s? t:f=w627:T31)
        n374 = property on="Compression" class="Slide (strict)"("DisabledEnum"=w627) -> ()  [unwired: 2 in, 2 out]
      }
      event "Tree": Double Click {
        n375 = event-data() -> ("PlatMods"=w637:T34, "Tag"=w636:string)  [unwired: 1 in]
        n376 = Unbundle(w637) -> ("Shift"=w635:bool)  [unwired: 4 out]
        n377 = Not(x=w635) -> (.not. x?=w634:bool)
        n378 = call <vilib>:"NT Update Persistence.vi"("Persistence"=w634, "Name"=w636) -> ()  [unwired: 9 in, 1 out]
      }
    }
  }
  n379 = local write "Dashboard Tab"(T2."Cool Stuff" ("Dashboard Tab")) -> ()
  n380 = property on="On/Off" class="Bool (strict)"("Visible"=w17) -> ()  [unwired: 2 in, 2 out]
  n381 = property on="Motor" class="Clust (strict)"("Visible"=w17) -> ()  [unwired: 2 in, 2 out]
  n382 = property on="Progress" class="Clust (strict)"("Visible"=w17) -> ()  [unwired: 2 in, 2 out]
  n383 = property on="Test Ring" class="Ring (strict)"("Visible"=w17) -> ()  [unwired: 2 in, 2 out]
  n384 = property on="Rev/Fwd" class="Clust (strict)"("Visible"=w17) -> ()  [unwired: 2 in, 2 out]
  n385 = property on="Camera Settings" class="Clust (strict)"("Visible"=w17) -> ()  [unwired: 2 in, 2 out]
  n386 = local write "DB Camera Config"(w17) -> ()
  n387 = while {
    tunnel: u16 1741 ("timeout ms (25000)") -> [w641]
    stop <- FALSE stop-if-true
    n388 = TCP Create Listener(10:w641) -> (0:w640:errorcluster, 3:w642:refnum<k5>)  [unwired: 4 in, 1 out]
    n389 = case shown="No Error" w640 {
      selector: w640 -> [w644 _]
      tunnel: w642 -> [w645 _]
      frame No Error {
        n390 = while {
          tunnel: w645 -> [w648]
          tunnel: w644 -> [w647]
          stop <- FALSE stop-if-true
          n391 = TCP Wait On Listener(8:w647, 11:w648) -> (0:w649:errorcluster, 4:w650:refnum<k5>)  [unwired: 2 in, 3 out]
          n392 = local write "TCP"(w650) -> ()
          n393 = case shown="No Error" w649 {
            frame No Error {
            }
            frame Error {
              n394 = Wait (ms)(milliseconds to wait=u32 1000) -> ()  [unwired: 1 out]
            }
          }
        }
      }
      frame Error {
        n395 = Wait (ms)(milliseconds to wait=u32 1000) -> ()  [unwired: 1 out]
      }
    }
  }
  n396 = local write "Command Params"(string[][] [] ("Command Params")) -> ()
  n397 = global write "WPI_DashboardLogging Global.vi" "Recording"(w43) -> ()
  n398 = local write "Command Selection"(u16 0 ("milliseconds to wait")) -> ()
  n399 = local write "Rec Mode"(w43) -> ()
